vi "NI 9215_READ.vi"(7 "Array":T1(array[cluster]) {"low cutoff freq: fl" format="%0.4f"}, 8 "error in (no error)":errorcluster, 9 "sampling freq: fs":dbl=1.0 format="%0.2f", 10 "number of samples per channel":i32=-1, 11 "Refnum in":refnum<k21>) -> (0 "error out":errorcluster, 1 "Filtered Value":dbl[](array[numeric]), 2 "Filtered (0-10V)":waveform(dbl)[](graph), 3 "Not Filtered (0-10V)":waveform(dbl)[](graph), 5 "task out":refnum<k21>)   [LabVIEW 2019]
uses:
  <vilib>/DAQmx/read.llb/DAQmx Read (Analog 1D Wfm NChan NSamp).vi
  <vilib>/Analysis/baseanly.llb/Mean (DBL).vi
  <vilib>/DAQmx/miscellaneous.llb/DAQmx Fill In Error Info.vi
  <vilib>/Analysis/NI_AALBase.lvlib
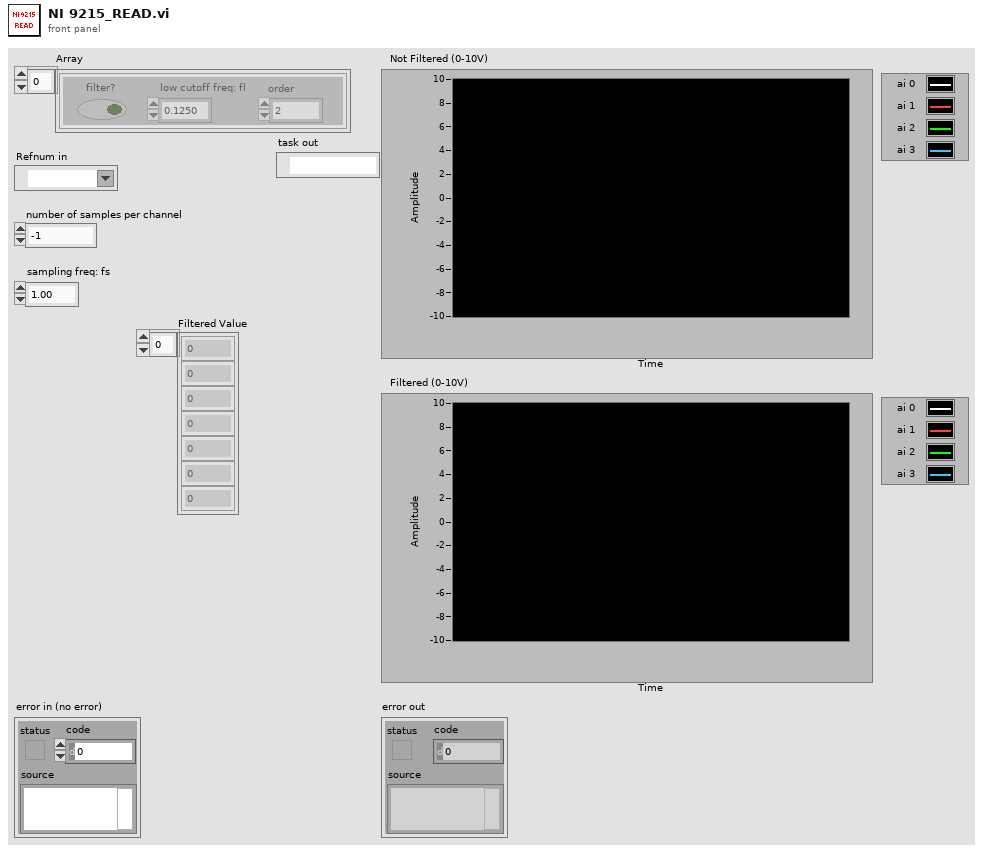
[diagram p1: front panel]
types:
  T1 = cluster{"filter?":bool, "low cutoff freq: fl":dbl, "order":i32}[]
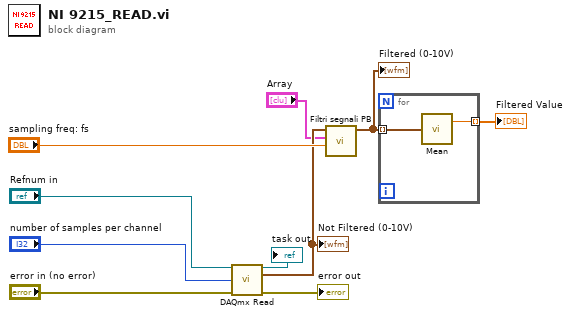
[diagram p0: block diagram]
diagram:
  n1 = call-poly <vilib>:"DAQmx Read.vi"("task/channels in"="Refnum in", "number of samples per channel"="number of samples per channel", "error in"="error in (no error)") -> ("task out"=→"task out":refnum<k21>, "data"=w6:waveform(dbl)[], "error out"=→"error out":errorcluster)  [unwired: 10 in]
  "Not Filtered (0-10V)" <- w6
  n2 = call "Filtri segnali PB.vi"("sampling freq: fs"="sampling freq: fs", "Array"="Array", "data in"=w6) -> ("filtered"=w2:waveform(dbl)[])  [unwired: 8 in]
  "Filtered (0-10V)" <- w2
  n3 = for {
    tunnel: [w12] -> w1 mode=indexing
    tunnel: w2 -> [w11] mode=indexing
    n4 = call-poly <vilib>:"Mean.vi"("X"=w11) -> ("mean"=w12:dbl)  [unwired: 1 out]
  }
  "Filtered Value" <- w1
